vi "SimpleMercuryiXXExample.vi"() -> ()   [LabVIEW 2014]
uses:
  <instrlib>/Mercury iXX/Public/Controls/Comms Transport Layer.ctl
  <instrlib>/Mercury iXX/Public/Controls/Serial Settings.ctl
  <instrlib>/Mercury iXX/Public/Controls/ISOBus Address.ctl
  <instrlib>/Mercury iXX/Public/Libraries/System/Open/Open System.vi
  <instrlib>/Mercury iXX/Public/Libraries/System/Read/Catalogue (Read).vi
  <instrlib>/Mercury iXX/Public/Libraries/System/Open/Open Device.vi
  <instrlib>/Mercury iXX/Public/Libraries/Temperature/Signals/Read/Temperature (Read).vi
  <instrlib>/Mercury iXX/Mercury iXX.lvlib
  <instrlib>/Mercury iXX/Public/Libraries/System.lvlib
  <instrlib>/Mercury iXX/Public/Libraries/Temperature.lvlib
panel:
  in  "IP Address":string="172.16.138.21"
  out "Temperature":dbl
  in  "Device Identifier":string="MB1.T1:TEMP"
  out "error out":errorcluster
  out "Catalogue of devices":string[](array[string])
  in  "ISOBUS address":T1=-1 caption="ISOBUS address (-1)"
  in  "ID Query (True)":bool
  in  "Serial Configuration":T2={"Baud Rate"=9600, "Parity"=0, "Data Bits"=8, "Stop Bits"=10, "Flow Control"=0} {"Flow Control" items=["None", "XON/XOFF", "RTS/CTS", "XON/XOFF & RTS/CTS", "DTR/DSR", "XON/XOFF & DTR/DSR"]; "Stop Bits" items=["1.0"=10, "2.0"=20]; "Data Bits" items=["7"=7, "8"=8]; "Parity" items=["None", "Odd", "Even"]; "Baud Rate" items=["300"=300, "600"=600, "1200"=1200, "2400"=2400, "4800"=4800, "9600"=9600, "19200"=19200]}
  in  "Comms Layer":T3
  in  "VISA resource name":refnum<visa-resource-name>="COM3"
  # "USB communication:\n1. Install the USB driver on your PC. (For a download\n   visit the mymercurysupport web site.)\n2. On the Settings screen of your Mercury Instrument:\n   a) General tab - set Remote Access to \"USB\" and\n      \"SCPI\" and apply the settings.\n   b) RS232 tab - make a note of the baud rate etc.\n3. On the Home screen, make sure that your Mercury\n   Instrument is in \"remote control\" mode (button at\n   bottom left is lit). \n4. Front panel controls to the right:\n   a) Comms Layer - \"USB\"\n   b) VISA resource name - click on the black arrow on\n      the right of the control and select the COM that\n      appeared after you installed the USB driver\n   c) Serial Configuration - enter baud rate etc to match\n      the data from 2b) above.\n5. Click on the white arrow above to run this VI.\n\nGPIB communication:\n1. On the Settings screen of your Mercury Instrument:\n   a) General tab - set Remote Access to \"GPIB\" and\n      \"SCPI\" and apply the settings.\n   b) GPIB tab - make a note of the GPIB address.\n2. On the Home screen, make sure that your Mercury\n   Instrument is in \"remote control\" mode (button at\n   bottom left is lit). \n3. Front panel controls to the right:\n   a) Comms Layer - \"GPIB\"\n   b) VISA resource name - click on the black arrow on\n      the right of the control and select the GPIB resource\n      with address that matches 1b) above.\n4. Click on the white arrow above to run this VI."
  # "Ethernet communication:\n1. On the Settings screen of your Mercury Instrument:\n   a) General tab - set Remote Access to \"Ethernet\" and\n      \"SCPI\" and apply the settings.\n   b) Ethernet tab - make a note of the IP address.\n2. On the Home screen, make sure that your Mercury\n   Instrument is in \"remote control\" mode (button at\n   bottom left is lit). \n3. Front panel controls to the right:\n   a) Comms Layer - \"Ethernet TCP/IP\"\n   b) IP Address  - enter the IP address from 1b) above\n4. Click on the white arrow above to run this VI.\n\nISOBus - RS-232 communication:\n1. On the Settings screen of your Mercury Instrument:\n   a) General tab - set Remote Access to \"ISOBUS\" and\n      \"SCPI\" and apply the settings.\n   b) ISOBUS tab - make a note of the ISOBUS address.\n      N.B. Each instrument connected to the ISOBUS\n           cable must have a different address\n   c) RS232 tab - make a note of the baud rate etc.\n2. On the Home screen, make sure that your Mercury\n   Instrument is in \"remote control\" mode (button at\n   bottom left is lit). \n3. Front panel controls to the right:\n   a) Comms Layer - \"ISOBus - RS-232\"\n   b) VISA resource name - click on the black arrow on\n      the right of the control and select the COM that\n      the ISOBUS cable is connected to.\n   c) ISOBUS address  - enter the address from 1b) above\n   d) Serial Configuration - enter baud rate etc to match\n      the data from 1c) above.\n4. Click on the white arrow above to run this VI."
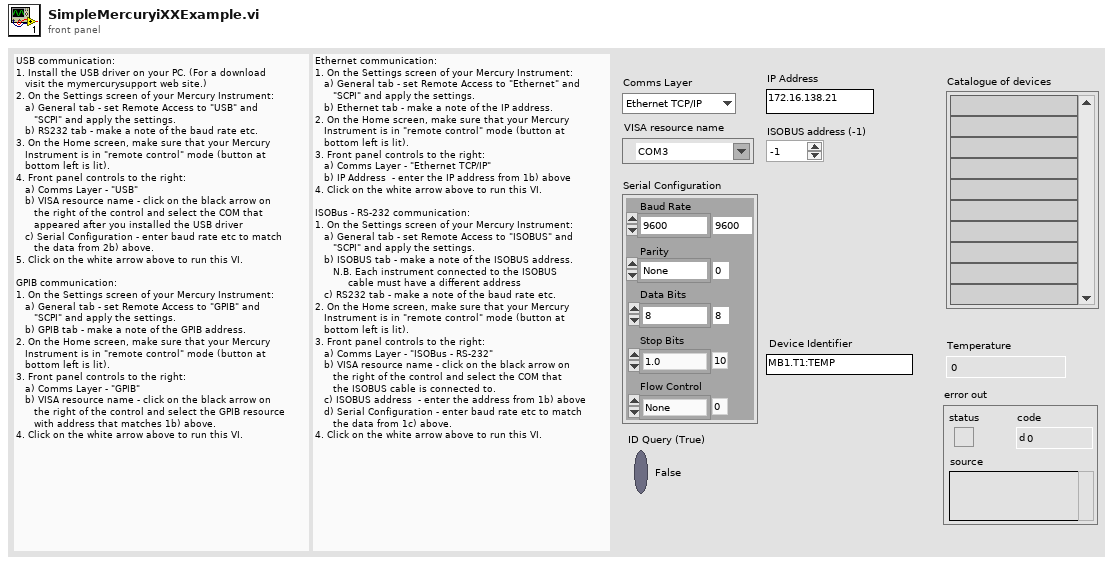
[diagram p1: front panel]
types:
  T1 = typedef "Mercury iXX.lvlib/ISOBus Address.ctl" = i32
  T2 = typedef "Mercury iXX.lvlib/Serial Settings.ctl" = cluster{"Baud Rate":u32, "Parity":u16, "Data Bits":u16, "Stop Bits":u16, "Flow Control":u16}
  T3 = typedef "Mercury iXX.lvlib/Comms Transport Layer.ctl" = enum16{"Ethernet TCP/IP", "USB", "ISOBus - RS-232", "GPIB"}
  T4 = typedef "Mercury iXX.lvlib/Mercury Reference.ctl" = cluster{"Comms":refnum<visa-resource-name>, "Device ID":string[], "Comms Layer":T3, "Command":string, "Query reference":T5}
  T5 = typedef "Mercury iXX.lvlib/Query Dynamic Reference.ctl" = refnum<vi>
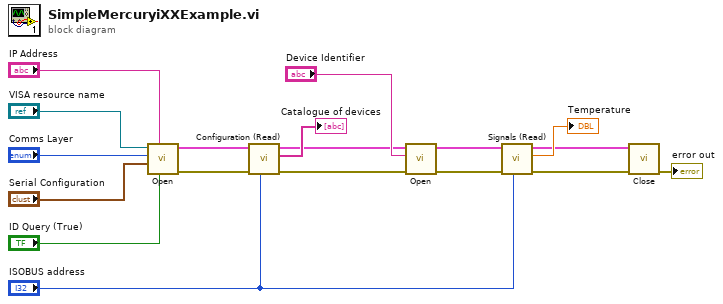
[diagram p0: block diagram]
diagram:
  n1 = call-poly <instrlib>:"Open.vi"("ID Query (True)"="ID Query (True)", "IP Address"="IP Address", "Serial Configuration"="Serial Configuration", "Comms Layer"="Comms Layer", "VISA resource name"="VISA resource name") -> ("error out"=w11:errorcluster, "Mercury Reference Out"=w12:T4)  [unwired: 2 in, 3 out]
  n2 = call-poly <instrlib>:"Configuration (Read).vi"("ISOBUS address"="ISOBUS address", "error in"=w11, "Mercury Reference In"=w12) -> ("error out"=w2:errorcluster, "Devices"=→"Catalogue of devices":string[], "Mercury Reference Out"=w3:T4)  [unwired: 5 in, 1 out]
  n3 = call-poly <instrlib>:"Open.vi"("error in (no error)"=w2, "Device Identifier"="Device Identifier", "Mercury Reference In"=w3) -> ("error out"=w8:errorcluster, "Mercury Reference Out"=w9:T4)  [unwired: 7 in]
  n4 = call-poly <instrlib>:"Signals (Read).vi"("ISOBUS address"="ISOBUS address", "error in"=w8, "Mercury Reference In"=w9) -> ("error out"=w4:errorcluster, "Temperature"=→"Temperature":dbl, "Mercury Reference Out"=w5:T4)  [unwired: 4 in, 2 out]
  n5 = call <instrlib>:"Close.vi"("error in (no error)"=w4, "Mercury Reference"=w5) -> ("error out"=→"error out":errorcluster)  [unwired: 9 in]
